vi "CANopen BatchSDO.vi"() -> ()   [LabVIEW 2016]
doc: "This example demonstrates how to write a batch SDO to a CANopen device."
uses:
  <vilib>/userdefined/High Color/nirio_resource_hc.ctl
  <vilib>/FPGAPlugInAG/cRIO-9033/niLvFpga_Open_cRIO-9033.vi
  <vilib>/rvi/interface/common/dynamic/niFpgaDynamicAddResources.vi
  <vilib>/CANopenLib/CANOPEN.llb/CANopen Interface Create.vi
  <vilib>/CANopenLib/CANOPEN.llb/CANopen SDO Create.vi
  <vilib>/CANopenLib/CANOPEN.llb/CANopen SDO Close.vi
  <vilib>/CANopenLib/CANOPEN.llb/CANopen Interface Close.vi
  <vilib>/FPGAPlugInAG/Dynamic/niLvFpga_Close_Dynamic.vi
  <vilib>/rvi/interface/nirviOpenFPGA/nirviOpenFPGA.xnode
  FPGA Bitfiles/project_FPGATarget_MainFPGA_S9ZLErdeBuw.lvbitx
  FPGA/MainFPGA.vi
  <vilib>/rvi/interface/nirviCloseFPGA/nirviCloseFPGA.xnode
panel:
  in  "error in":errorcluster
  out "completion code":u32 format="%.0x"
  in  "batch SDO name":string="BatchSDO"
  in  "node-ID":u8=1 min=1 max=127 step=1
  in  "baud rate":u32(ring)=2 items=["1 Mbit/s"=0, "800 kbit/s"=1, "500 kbit/s"=2, "250 kbit/s"=3, "125 kbit/s"=4, "50 kbit/s"=6, "20 kbit/s"=7, "10 kbit/s"=8]
  in  "CANopen interface":u32(ring) items=["CANopen01", "CANopen02", "CANopen03", "CANopen04", "CANopen05", "CANopen06", "CANopen07", "CANopen08", "CANopen09", "CANopen10", "CANopen11", "CANopen12", "CANopen13", "CANopen14", "CANopen15", "CANopen16", "CANopen17", "CANopen18", "CANopen19", "CANopen20", "CANopen21", "CANopen22", "CANopen23", "CANopen24", "CANopen25", "CANopen26", "CANopen27", "CANopen28", "CANopen29", "CANopen30", "CANopen31", "CANopen32"]
  # "Overview: This example demonstrates how to write a Batch SDO to a CANopen device.\nRequirements: Connect CANopen module with a slave device.\nInstructions:\n1. In NI CANopen for PXI PCI project, right-click My Computer or RT Target and select New»CANopen Batch SDO from the shortcut\n    menu. Specify the device name in the BatchSDO dialog box that appears and click OK. \n2. In this dialog box, click the Object Dictionary tab and add the items to use for Batch SDO.\n3. Click the Batch SDO Preview tab and click the Generate Batch SDO Preview to preview batch SDO.\n4. Click the Online Validation tab, configure the settings and click Send Batch SDO to validate batch SDO. Click OK.\n5. Right-click the BatchSDO item that you create and select Deploy from the shortcut menu. \n6. Specify the values of CANopen interface, baud rate of the CANopen interface and node-ID of the slave device.\n7. Set batch SDO name the same as the name of batch SDO under the same target.\n8. Run this VI to send SDOs to CANopen device."
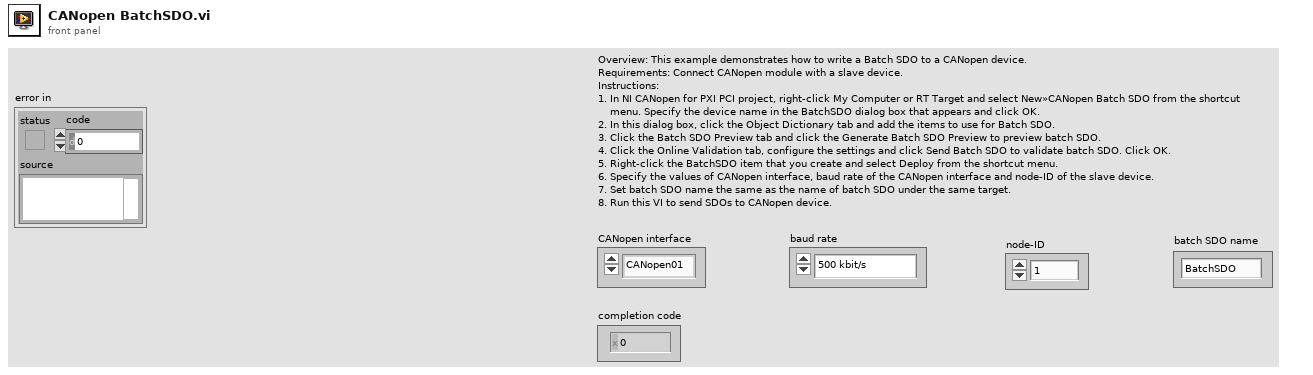
[diagram p1: front panel]
types:
  T1 = typedef "nirio_resource_hc.ctl" = tag
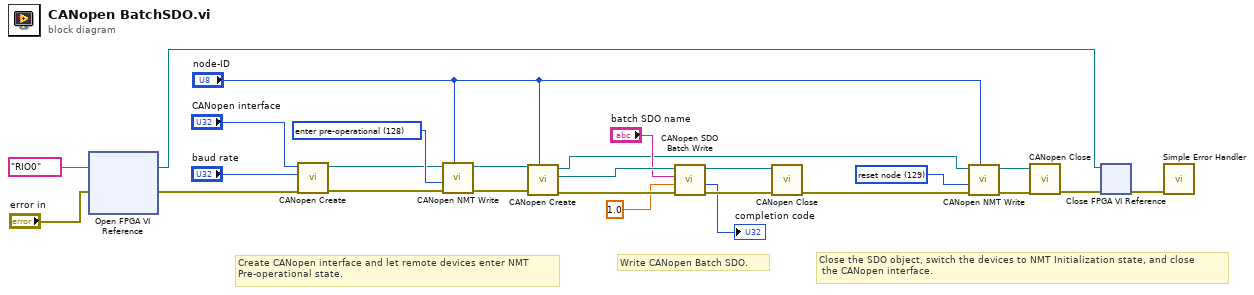
[diagram p0: block diagram]
diagram:
  w11 = u16 129 items=["start remote node"=1, "stop remote node"=2, "enter pre-operational"=128, "reset node"=129, "reset communication"=130] ("command")
  w22 = u16 128 items=["start remote node"=1, "stop remote node"=2, "enter pre-operational"=128, "reset node"=129, "reset communication"=130] ("command")
  # "Close the SDO object, switch the devices to NMT Initialization state, and close\n the CANopen interface."
  # "Create CANopen interface and let remote devices enter NMT\nPre-operational state."
  # "Write CANopen Batch SDO."
  n1 = xnode ("Open FPGA VI Reference")("error in"="error in", "resource name"=T1 "RIO0") -> ("FPGA VI Reference Out"=w1:refnum<k20>, "error out"=w4:errorcluster)
  n2 = call-poly <vilib>:"CANopen Create.vi"("error in (no error)"=w4, "baud rate"="baud rate", "interface name"="CANopen interface") -> ("error out"=w21:errorcluster, "interface object out"=w20:refnum<k20>)  [unwired: 7 in]
  n3 = call <vilib>:"CANopen NMT Write.vi"("node-ID (0)"="node-ID", "error in (no error)"=w21, "command"=w22, "interface object in"=w20) -> ("error out"=w25:errorcluster, "interface object out"=w26:refnum<k20>)  [unwired: 6 in]
  n4 = call-poly <vilib>:"CANopen Create.vi"("node-ID"="node-ID", "error in (no error)"=w25, "interface object in"=w26) -> ("error out"=w18:errorcluster, "SDO object out"=w19:refnum<k20>, "interface object out"=w8:refnum<k20>)  [unwired: 6 in]
  n5 = call <vilib>:"CANopen SDO Batch Write.vi"("error in (no error)"=w18, "timeout (1s)"=1.0 ("timeout (0s)"), "batch SDO name"="batch SDO name", "SDO object in"=w19) -> ("error out"=w16:errorcluster, "completion code"=→"completion code":u32, "SDO object out"=w15:refnum<k20>)  [unwired: 5 in]
  n6 = call-poly <vilib>:"CANopen Close.vi"("error in (no error)"=w16, "SDO object in"=w15) -> ("error out"=w12:errorcluster)  [unwired: 9 in]
  n7 = call <vilib>:"CANopen NMT Write.vi"("node-ID (0)"="node-ID", "error in (no error)"=w12, "command"=w11, "interface object in"=w8) -> ("error out"=w10:errorcluster, "interface object out"=w9:refnum<k20>)  [unwired: 6 in]
  n8 = call-poly <vilib>:"CANopen Close.vi"("error in (no error)"=w10, "interface object in"=w9) -> ("error out"=w3:errorcluster)  [unwired: 9 in]
  n9 = xnode "Close FPGA VI Reference"("FPGA VI Reference In"=w1, "error in"=w3) -> ("error out"=w2:errorcluster)
  n10 = call <vilib>:"Simple Error Handler.vi"("error in (no error)"=w2) -> ()  [unwired: 4 in, 5 out]
